vi "ReadVoltage_HT.vi"(6 "error in (no error)":errorcluster, 9 "Voltage to Measure":string(combo)="Bandgap") -> (0 "error out":errorcluster, 3 "Voltage Read":dbl)   [LabVIEW 2011]
doc: "This VI reads a chosen voltage of a NB PLL.\n\nInputs:\n1. Voltage to Measure: Selects the voltage that will be read by the SRP ADC (ie. BG, VA, VD, etc.).\n\nOutputs:\n1.Voltage Read: The value of the chosen measurement in volts."
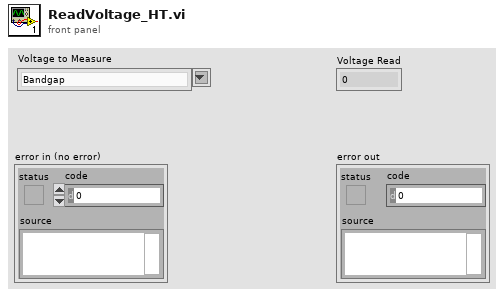
[diagram p1: front panel]
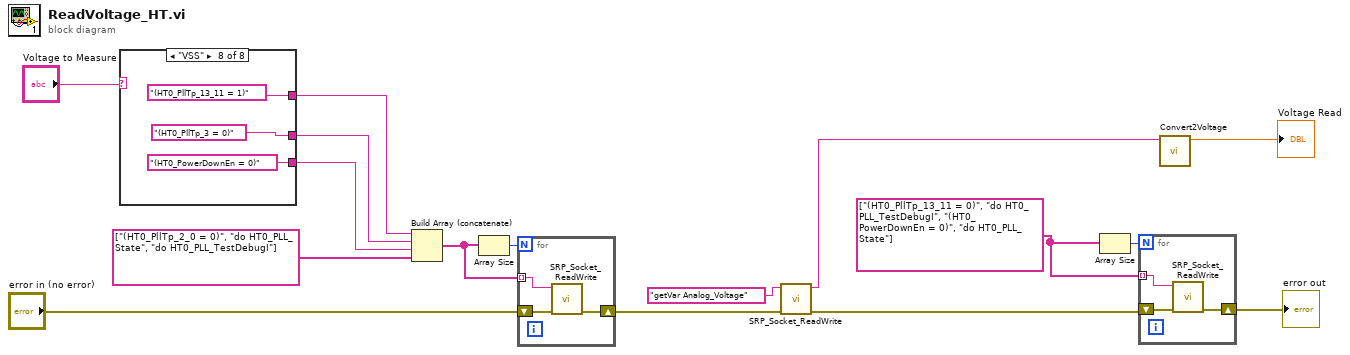
[diagram p0: block diagram]
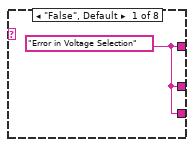
[diagram p2: hidden frame]
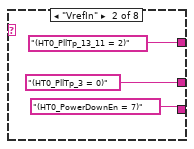
[diagram p3: hidden frame]
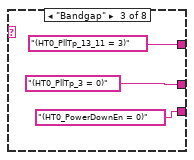
[diagram p4: hidden frame]
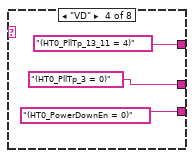
[diagram p5: hidden frame]
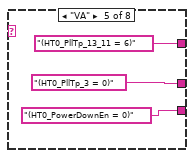
[diagram p6: hidden frame]
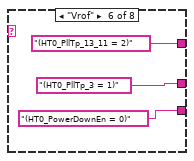
[diagram p7: hidden frame]
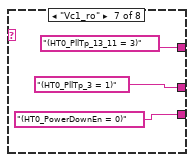
[diagram p8: hidden frame]
diagram:
  w3 = string[] ["(HT0_PllTp_13_11 = 0)", "do HT0_PLL_TestDebugI", "(HT0_PowerDownEn = 0)", "do HT0_PLL_State"]
  n1 = case shown="\"VSS\"" "Voltage to Measure" {
    tunnel: [w17 "(HT0_PllTp_13_11 = 2)" "(HT0_PllTp_13_11 = 3)" "(HT0_PllTp_13_11 = 4)" "(HT0_PllTp_13_11 = 6)" "(HT0_PllTp_13_11 = 2)" "(HT0_PllTp_13_11 = 3)" "(HT0_PllTp_13_11 = 1)"] -> w15
    tunnel: [w17 "(HT0_PllTp_3 = 0)" "(HT0_PllTp_3 = 0)" "(HT0_PllTp_3 = 0)" "(HT0_PllTp_3 = 0)" "(HT0_PllTp_3 = 1)" "(HT0_PllTp_3 = 1)" "(HT0_PllTp_3 = 0)"] -> w12
    tunnel: [w17 "(HT0_PowerDownEn = 7)" "(HT0_PowerDownEn = 0)" "(HT0_PowerDownEn = 0)" "(HT0_PowerDownEn = 0)" "(HT0_PowerDownEn = 0)" "(HT0_PowerDownEn = 0)" "(HT0_PowerDownEn = 0)"] -> w11
    frame "False", Default {
      w17 = "Error in Voltage Selection"
    }
    frame "VrefIn" {
    }
    frame "Bandgap" {
    }
    frame "VD" {
    }
    frame "VA" {
    }
    frame "Vrof" {
    }
    frame "Vc1_ro" {
    }
    frame "VSS" {
    }
  }
  n2 = Build Array (concatenate)(w15, w12, w11, string[] ["(HT0_PllTp_2_0 = 0)", "do HT0_PLL_State", "do HT0_PLL_TestDebugI"]) -> (w14:string[])
  n3 = Array Size(array=w14) -> (size(s)=w13:i32)
  n4 = for {
    N: w13 -> [_]
    tunnel: w14 -> [w39] mode=indexing
    shift-right: [w40] -> w10
    shift-left: "error in (no error)" -> [w41]
    n5 = call "SRP_Socket_ReadWrite.vi"("error in (no error)"=w41, "Data In"=w39) -> ("error out"=w40:errorcluster)  [unwired: 7 in, 1 out]
  }
  n6 = call "SRP_Socket_ReadWrite.vi"("error in (no error)"=w10, "Data In"="getVar Analog_Voltage") -> ("error out"=w2:errorcluster, "Data Out"=w6:string)  [unwired: 7 in]
  n7 = Array Size(array=w3) -> (size(s)=w4:i32)
  n8 = for {
    N: w4 -> [_]
    tunnel: w3 -> [w42] mode=indexing
    shift-right: [w43] -> w1
    shift-left: w2 -> [w44]
    n9 = call "SRP_Socket_ReadWrite.vi"("error in (no error)"=w44, "Data In"=w42) -> ("error out"=w43:errorcluster)  [unwired: 7 in, 1 out]
  }
  "error out" <- w1
  n10 = call "Convert2Voltage.vi"("SRP ADC String"=w6) -> ("Voltage"=→"Voltage Read":dbl)  [unwired: 10 in]
